vi "Initialize (Local).vi"(0 "device":refnum<k21>, 1 "topology suffix (none)":string, 5 "Topology":string, 9 "reset device (boolean value)":bool=TRUE, 11 "error in (no error)":errorcluster) -> (4 "SLSC Switch out":refnum<class "SLSC Switch.lvclass">, 15 "error out":errorcluster)   [LabVIEW 2016, in "SLSC Switch.lvlib" / "SLSC Switch.lvclass"]
doc: "Returns a session handle used to identify the switch module in all subsequent driver calls and sets the topology of the switch module."
uses:
  SLSC Switch.lvclass
  <vilib>/National Instruments/SLSC Local or Remote Interface/SLSC Local Interface Class/SLSC Local.lvclass
  C:/Program Files (x86)/National Instruments/LabVIEW 2016/vi.lib/National Instruments/SLSC Local or Remote Interface/SLSC Interface Class/SLSC Interface.lvclass
  <vilib>/National Instruments/SLSC Local or Remote Interface/SLSC Local Interface Class/Initialize (NVMEM Area).vi
  <vilib>/National Instruments/SLSC Local or Remote Interface/SLSC Local Interface Class/Initialize (No Resource).vi
  <vilib>/National Instruments/SLSC Local or Remote Interface/SLSC Interface Class/SLSC Interface.lvclass
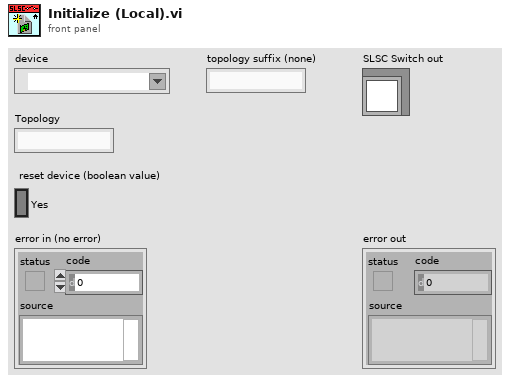
[diagram p1: front panel]
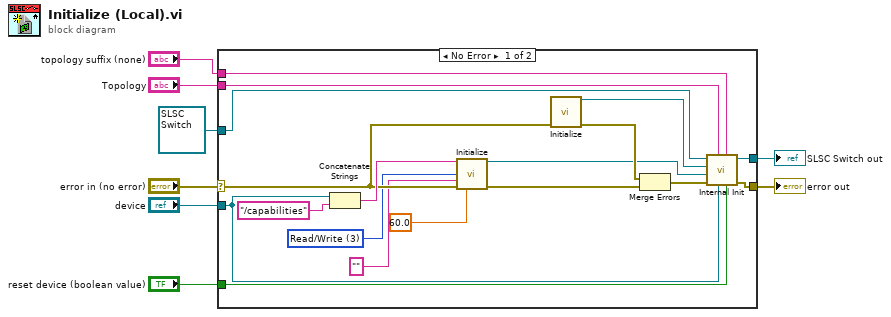
[diagram p0: block diagram]
diagram:
  n1 = case shown="No Error" "error in (no error)" {
    selector: "error in (no error)" -> [w19 w28]
    tunnel: [w25 w28] -> w7
    tunnel: refnum<class "SLSC Switch.lvclass"> refnum ("SLSC Switch in") -> [w26 w27]
    tunnel: "device" -> [w21 _]
    tunnel: "Topology" -> [w12 _]
    tunnel: "reset device (boolean value)" -> [w13 _]
    tunnel: [w24 w27] -> w2
    tunnel: "topology suffix (none)" -> [w23 _]
    frame No Error {
      w11 = 3 items=["None"=0, "Read Only"=1, "Read/Write"=3] ("reservation access (Read/Write)")
      n2 = Concatenate Strings(w21, "/capabilities" ("string")) -> (w20:string)
      n3 = call-poly <vilib>:"Initialize.vi"("NVMEM areas"=w20, "reservation access (Read/Write)"=w11, "reservation group"="", "error in (no error)"=w19, "connect timeout (60 sec)"=60.0) -> ("SLSC Local out"=w15:refnum<class "SLSC Local.lvclass">, "error out"=w17:errorcluster)  [unwired: 9 in]
      n4 = call-poly <vilib>:"Initialize.vi"("error in (no error)"=w19) -> ("SLSC Local out"=w14:refnum<class "SLSC Local.lvclass">, "error out"=w18:errorcluster)  [unwired: 13 in]
      n5 = Merge Errors(w18, w17) -> (w16:errorcluster)
      n6 = call "Internal Init.vi"("reset device (boolean value)"=w13, "topology suffix (none)"=w23, "device"=w21, "Topology"=w12, "error in (no error)"=w16, "NVMEM Session"=w15, "No Resource Session"=w14, "SLSC Switch in"=w26) -> ("error out"=w25:errorcluster, "SLSC Switch out"=w24:refnum<class "SLSC Switch.lvclass">)  [unwired: 2 in]
    }
    frame Error {
    }
  }
  "error out" <- w7
  "SLSC Switch out" <- w2
